vi "Read timeData.vi"(8 "error in":errorcluster, 11 "PAS Cell Data in":refnum<class "PAS Cell Data.lvclass">) -> (0 "error out":errorcluster, 2 "timeData":waveform(i16), 3 "PAS Cell Data out":refnum<class "PAS Cell Data.lvclass">)   [LabVIEW 2014, in "PAS Cell Data.lvclass"]
uses:
  PAS Cell Data.lvclass
  PAS Cell Data.lvclass/PAS Cell Data.ctl
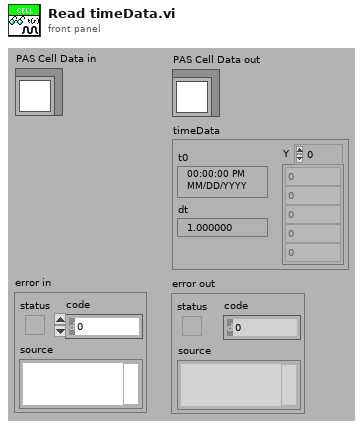
[diagram p1: front panel]
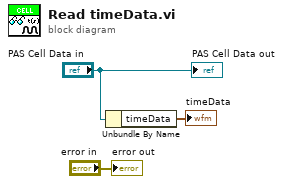
[diagram p0: block diagram]
diagram:
  n1 = Unbundle By Name("PAS Cell Data in") -> ("timeData"=→"timeData":waveform(i16))
  "error out" <- "error in"
  "PAS Cell Data out" <- "PAS Cell Data in"
